vi "xiC - IMAQ - PLAY.vi"(6 "Data":variant, 8 "error in (no error)":errorcluster, 11 "Attributes In":T1) -> (0 "error out":errorcluster, 3 "Attributes In":T1)   [LabVIEW 2015]
uses:
  C:/GIT/Cameras3.x/Integrations/Labview/xiLib/xiLIB_32bit/xiLIB/xiCamLib/API/x86/xiApi.NET.dll
  xiLIB_32bit/xiLIB/xiCamLib/API/x86/xiApi.NET.dll
  <vilib>/vision/Image Controls.llb/IMAQ Image.ctl
  xiC - IMAQ - TreeDisplayType.ctl
  xiC - IMAQ - Attributes.ctl
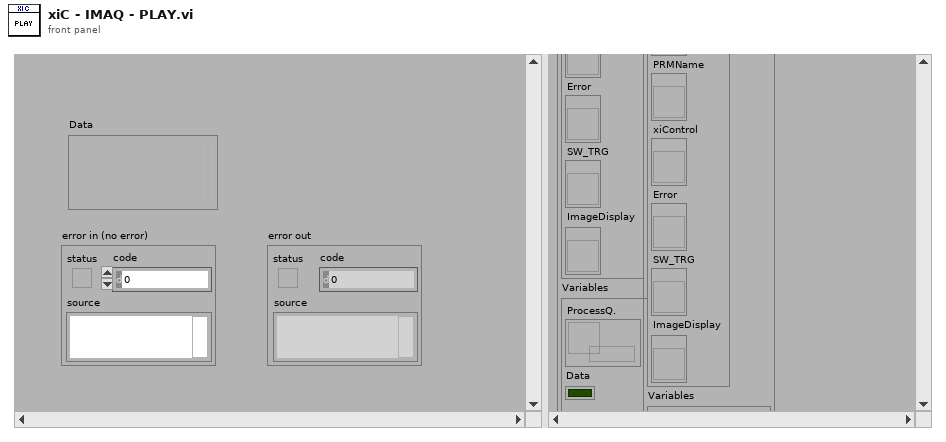
[diagram p1: front panel]
types:
  T1 = typedef "xiC - IMAQ - Attributes.ctl" = cluster{"Controls":cluster{"VI Ref.":refnum<vi>, "Tree":refnum<vi>, "Info":refnum<vi>, "PRMName":refnum<vi>, "xiControl":refnum<vi>, "Error":refnum<vi>, "SW_TRG":refnum<vi>, "ImageDisplay":refnum<vi>}, "Variables":cluster{"ProcessQ.":refnum<queue>, "Data":bool, "xiCam":refnum<k24>, "Tree_Display_Type":T2}}
  T2 = typedef "xiC - IMAQ - TreeDisplayType.ctl" = enum16{"DEFAULT", "HIDE_MAX_MIN"}
  T3 = typedef "IMAQ Image.ctl" = refnum<image>
  T4 = typedef "xiImageMng - Attributes.ctl" = cluster{"WIDTH":i32, "HEIGHT":i32, "IMG_FORMAT":T5}
  T5 = typedef "IMG_DATA_FORMAT.ctl" = enum16{"MONO8", "MONO16", "RGB24", "RGB32", "RGBPLANAR", "RAW8", "RAW16"}
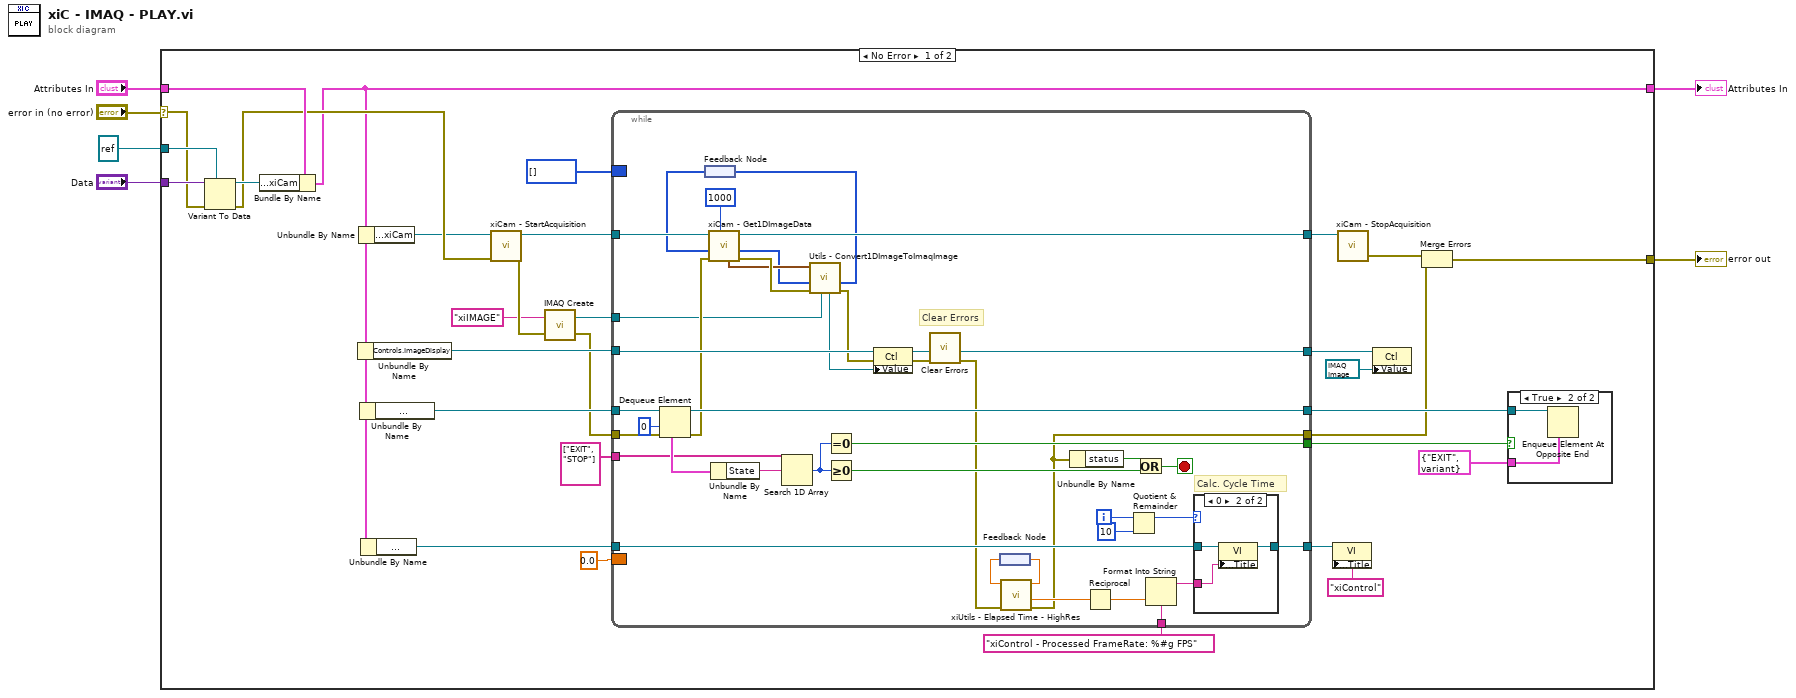
[diagram p0: block diagram]
diagram:
  n1 = case shown="No Error" "error in (no error)" {
    selector: "error in (no error)" -> [w16 w85]
    tunnel: [w24 w85] -> w6
    tunnel: "Attributes In" -> [w17 w84]
    tunnel: [w14 w84] -> w4
    tunnel: "Data" -> [w20 _]
    tunnel: refnum<k24> refnum ("Variables.xiCam") -> [w19 _]
    frame No Error {
      n2 = Variant To Data(error in=w16, type=w19, Variant=w20) -> (data=w18:refnum<k24>, error out=w15:errorcluster)
      n3 = Bundle By Name(cluster=w17, "Variables.xiCam"=w18) -> (w14:T1)
      n4 = Unbundle By Name(w14) -> ("Controls.ImageDisplay"=w28:refnum<vi>)
      n5 = Unbundle By Name(w14) -> ("Variables.xiCam"=w13:refnum<k24>)
      n6 = Unbundle By Name(w14) -> ("Variables.ProcessQ."=w37:refnum<queue>)
      n7 = Unbundle By Name(w14) -> ("Controls.VI Ref."=w31:refnum<vi>)
      n8 = call "xiCam - StartAcquisition.vi"("error in (no error)"=w15, "xiCam In"=w13) -> ("error out"=w12:errorcluster, "xiCam Out"=w29:refnum<k24>)  [unwired: 8 in]
      n9 = call "IMAQ Create"("Image Name"="xiIMAGE", "error in (no error)"=w12) -> ("New Image"=w10:T3, "error out"=w11:errorcluster)  [unwired: 3 in]
      n10 = while {
        tunnel: w37 -> [w79]
        tunnel: w11 -> [w78]
        tunnel: string[] ["EXIT", "STOP"] -> [w74]
        tunnel: [w50] -> w25
        tunnel: [w70] -> w35
        tunnel: [w69] -> w34
        border: 0.0 ("Tick (ms) In") -> [_]
        tunnel: w31 -> [w60]
        tunnel: "xiControl - Processed FrameRate: %#g FPS" ("format string") -> [w62]
        border: u8[] [] -> [_]
        tunnel: w29 -> [w58]
        tunnel: [w56] -> w27
        tunnel: w28 -> [w55]
        tunnel: [w54] -> w23
        tunnel: [w53] -> w22
        tunnel: w10 -> [w45]
        i -> [w65]
        stop <- w72 stop-if-true
        # "Clear Errors"
        # "Calc. Cycle Time"
        n11 = Dequeue Element(queue=w79, timeout in ms (-1)=0, error in (no error)=w78) -> (queue out=w69:refnum<queue>, element=w76:cluster{"State":string, "Data":variant}, error out=w51:errorcluster)  [unwired: 1 out]
        n12 = feedback #1() -> (w57:u8[])
        n13 = call "xiCam - Get1DImageData.vi"("timeout"=1000, "error in (no error)"=w51, "1DImageData In"=w57, "xiCam In"=w58) -> ("error out"=w49:errorcluster, "1DImageData Out"=w42:u8[], "xiCam Out"=w56:refnum<k24>, "Image Properites"=w46:T4)  [unwired: 4 in]
        n14 = Unbundle By Name(w76) -> ("State"=w75:string)
        n15 = Search 1D Array(1D array=w74, element=w75) -> (index of element=w71:i32)  [unwired: 1 in]
        n16 = call "Utils - Convert1DImageToImaqImage.vi"("Image In"=w45, "error in (no error)"=w49, "1DImageData In"=w42, "Image Properties In"=w46) -> ("error out"=w43:errorcluster, "1DImageData Out"=w48:u8[], "Image Out"=w44:T3)  [unwired: 5 in]
        n17 = feedback-in #1(w48) -> ()
        n18 = Equal To 0?(x=w71) -> (x = 0?=w70:bool)
        n19 = Greater Or Equal To 0?(x=w71) -> (x >= 0?=w73:bool)
        n20 = property class="Ctl"(reference=w55, error in=w43, "Value"=w44) -> (reference out=w54:refnum<vi>, error out=w41:errorcluster)
        n21 = call <vilib>:"Clear Errors.vi"("error in (no error)"=w41) -> ("error out"=w40:errorcluster)  [unwired: 5 in, 1 out]
        n22 = feedback #2() -> (w67:dbl)
        n23 = call "xiUtils - Elapsed Time - HighRes.vi"("error in (no error)"=w40, "Tick (ms) In"=w67) -> ("error out"=w50:errorcluster, "Elapsed Time(ms)"=w63:dbl, "Tick (ms) Out"=w68:dbl)  [unwired: 7 in]
        n24 = feedback-in #2(w68) -> ()
        n25 = Unbundle By Name(w50) -> ("status"=w59:bool)
        n26 = Reciprocal(x=w63) -> (1/x=w47:dbl)
        n27 = Quotient & Remainder(x=w65, y=10) -> (x-y*floor(x/y)=w64:i32)  [unwired: 1 out]
        n28 = Or(x=w59, y=w73) -> (x .or. y?=w72:bool)
        n29 = Format Into String(format string=w62, w47) -> (resulting string=w61:string)  [unwired: 2 in, 1 out]
        n30 = case shown="0" w64 {
          tunnel: w61 -> [_ w82]
          tunnel: w60 -> [w80 w83]
          tunnel: [w80 w81] -> w53
          frame Default {
          }
          frame 0 {
            n31 = property class="VI"(reference=w83, "Front Panel.Title"=w82) -> (reference out=w81:refnum<vi>)  [unwired: 1 in, 1 out]
          }
        }
      }
      n32 = property class="VI"(reference=w22, "Front Panel.Title"="xiControl" ("format string")) -> ()  [unwired: 1 in, 2 out]
      n33 = call "xiCam - StopAcquisition.vi"("xiCam In"=w27) -> ("error out"=w26:errorcluster)  [unwired: 9 in, 1 out]
      n34 = property class="Ctl"(reference=w23, "Value"=T3 refnum ("New Image")) -> ()  [unwired: 1 in, 2 out]
      n35 = Merge Errors(w26, w25) -> (w24:errorcluster)
      n36 = case shown="True" w35 {
        tunnel: w34 -> [_ w39]
        tunnel: cluster{"State":string, "Data":variant} {"State"="EXIT", "Data"=variant} ("element") -> [_ w38]
        frame False {
        }
        frame True {
          n37 = Enqueue Element At Opposite End(queue=w39, element=w38) -> ()  [unwired: 2 in, 3 out]
        }
      }
    }
    frame Error {
    }
  }
  "error out" <- w6
  "Attributes In" <- w4
